vi "xcamera-make_trigger-source-frame-start.vi"(11 "Option":T1(ring)) -> (3 "Serial String":string)   [LabVIEW 2012]
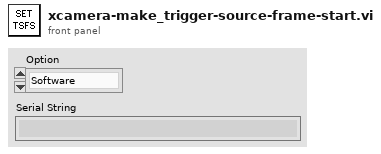
[diagram p1: front panel]
types:
  T1 = enum16{"Software", "Line1", "Line2", "CC1", "CC2", "CC3", "CC4"}
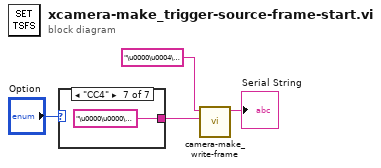
[diagram p0: block diagram]
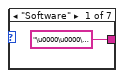
[diagram p2: hidden frame]
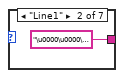
[diagram p3: hidden frame]
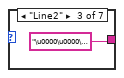
[diagram p4: hidden frame]
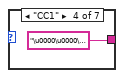
[diagram p5: hidden frame]
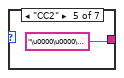
[diagram p6: hidden frame]
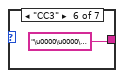
[diagram p7: hidden frame]
diagram:
  n1 = case shown="\"CC4\"" "Option" {
    tunnel: ["\u0000\u0000\u0000\u0000" ("Address") "\u0000\u0000\u0000\u0001" ("Address") "\u0000\u0000\u0000\u0001" ("Address") "\u0000\u0000\u0000\t" ("Address") "\u0000\u0000\u0000\n" ("Address") "\u0000\u0000\u0000\u000b" ("Address") "\u0000\u0000\u0000\f" ("Address")] -> w1
    frame "Software" {
    }
    frame "Line1" {
    }
    frame "Line2" {
    }
    frame "CC1" {
    }
    frame "CC2" {
    }
    frame "CC3" {
    }
    frame "CC4" {
    }
  }
  n2 = call "camera-make_write-frame.vi"("Data"=w1, "Address"="\u0000\u0004\u0002@") -> ("Serial String"=→"Serial String":string)  [unwired: 9 in]
